vi "Find_or_Set_Creator_Type.vi"() -> ()   [LabVIEW 2010]
panel:
  in  "Mode":enum16{"Single File", "All Files inside Folder"}(ring)
  in  "new creator":string="XCEL"
  in  "Set creater type":bool
  out "Current creator":string
  out "Path":path
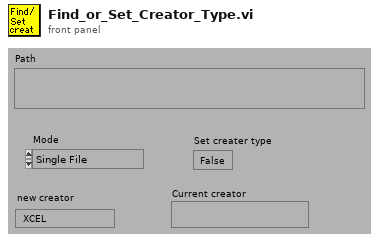
[diagram p1: front panel]
types:
  T1 = enum32{"existing file", "new file", "new or existing file", "existing dir", "new dir", "new or existing dir", "existing file (use LLBs)", "new file (use LLBs)", "new or existing file (use LLBs)", "new or existing file or directory (use LLBs)"}
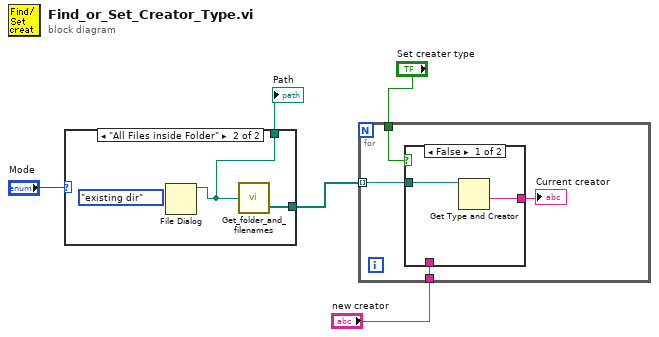
[diagram p0: block diagram]
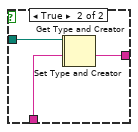
[diagram p2: hidden frame]
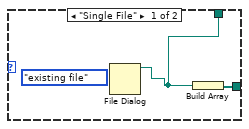
[diagram p3: hidden frame]
diagram:
  n1 = case shown="\"All Files inside Folder\"" "Mode" {
    tunnel: [w7 w9] -> w2
    tunnel: [w6 w8] -> w1
    frame "Single File" {
      (unwired) T1."existing file" ("select mode (2)")
      n2 = File Dialog() -> (3:w6:path)  [unwired: 7 in, 3 out]
      n3 = Build Array(w6) -> (w7:path[])
    }
    frame "All Files inside Folder" {
      (unwired) T1."existing dir" ("select mode (2)")
      n4 = File Dialog() -> (3:w8:path)  [unwired: 7 in, 3 out]
      n5 = call "Get_folder_and_filenames.vi"("file path (dialog if empty)"=w8) -> ("Files"=w9:path[])  [unwired: 1 out]
    }
  }
  "Path" <- w1
  n6 = for {
    tunnel: "Set creater type" -> [w13]
    tunnel: "new creator" -> [w12]
    tunnel: w2 -> [w11] mode=indexing
    n7 = case shown="False" w13 {
      tunnel: w11 -> [w15 w20]
      tunnel: [w14 w19] -> w10
      tunnel: w12 -> [_ w18]
      frame False {
        n8 = Get Type and Creator(7:w15) -> (1:w14:string)  [unwired: 1 in, 3 out]
      }
      frame True {
        n9 = Set Type and Creator(5:w18, 7:w20) -> (0:w16:errorcluster, 3:w17:path)  [unwired: 2 in]
        n10 = Get Type and Creator(4:w16, 7:w17) -> (1:w19:string)  [unwired: 3 out]
      }
    }
    "Current creator" <- w10
  }
